vi "Vision Server Get Timestamp.vi"() -> (0 "Timestamp (ms)":dbl)   [LabVIEW 2016]
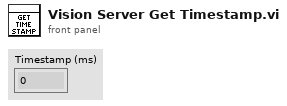
[diagram p1: front panel]
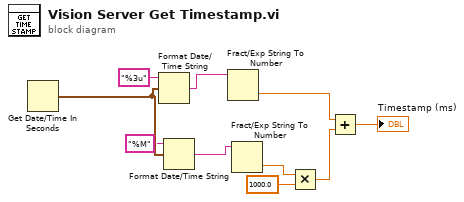
[diagram p0: block diagram]
diagram:
  n1 = Get Date/Time In Seconds() -> (seconds since 1Jan1904=w9:timestamp)
  n2 = Format Date/Time String(time format string (%c)="%3u", seconds (now)=w9) -> (date/time string=w7:string)  [unwired: 1 in]
  n3 = Format Date/Time String(time format string (%c)="%M", seconds (now)=w9) -> (date/time string=w6:string)  [unwired: 1 in]
  n4 = Fract/Exp String To Number(string=w7) -> (number=w3:dbl)  [unwired: 3 in, 1 out]
  n5 = Fract/Exp String To Number(string=w6) -> (number=w5:dbl)  [unwired: 3 in, 1 out]
  n6 = Multiply(x=w5, y=1000.0) -> (x*y=w2:dbl)
  n7 = Add(x=w3, y=w2) -> (x+y=→"Timestamp (ms)":dbl)
